vi "AlliGator Save-Load Settings.vi"(6 "Load(F)/Save (T)":bool, 8 "Error In":errorcluster, 10 "File Path":path, 11 "AlliGator Refnum in":refnum<vi>) -> (0 "Error Out":errorcluster, 2 "File Path out":path)   [LabVIEW 2021, in "AlliGator Settings.lvlib"]
doc: "Use this file to Save or Load AlliGator's settings to an ini file.\n\nIf the <B>File Path</B> input is left unconnected, the defaut ini file is used (overriding the current ini file).\n\nTo save settings in a user-specified location, either provide a valid path, or connect a \"Not a Path\" constant to the input. A File Dialog window will then open to allow the user to choose a path."
uses:
  AlliGator Settings.lvlib
  AlliGator Settings List.ctl
  <vilib>/Utility/sysdir.llb/System Directory Type.ctl
  97c900eb-8bb6-49ac-a854-86d526cd6a68.vi
  97c900eb-8bb6-49ac-a854-86d526cd6a68.vi/539bd7ec-d9e8-460f-a56d-a449b4a86a5e.vi
  Files/Files.lvlib
  <vilib>/Utility/config.llb/NI_LVConfig.lvlib
  <userlib>/_OpenG.lib/variantconfig/variantconfig.llb/openg_variant_configuration_file.lvlib
  Strings/Strings.lvlib
  Graphs/Graphs.lvlib
panel:
  in  "AlliGator Settings List":T1
  # "see the AlliGator License on the block diagram (Ctrl+E or Window:Show Block Diagram)"
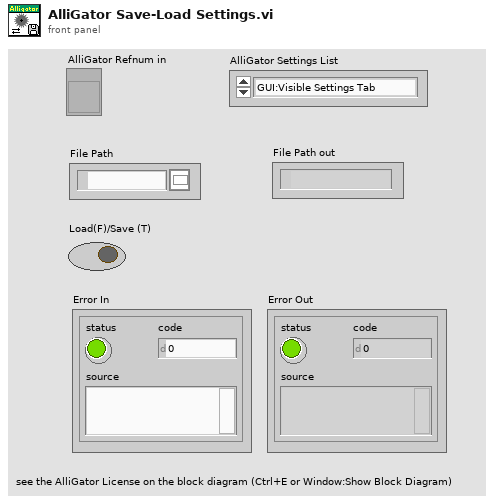
[diagram p1: front panel]
types:
  T1 = typedef "AlliGator Settings.lvlib/AlliGator Settings List.ctl" = enum16{"GUI:Visible Settings Tab", "GUI:Last Run Version", "Source Image:Use Image Histogram for Contrast", "Source Image:Low Count Pixels Rejection Options", "Source Image:High Count Pixels Rejection Options", "Source Image:Use Image Brightness", "Source Image:Blend Overlay with Image Background", "Source Image:Use Fixed ROI Diameter", "Source Image:ROI Diameter", "Source Image:ROI Center Color", "Source Image:Peak Threshold", "Source Image:Intensity Threshold", "Source Image:Image Binning Options", "Source Image:Image Smoothing Options", "Source Image:Image Histogram Active", "Source Image:Invert Binary Mask", "Source Image:Hot Pixel Removal", "Source Image:Overlay Analyzed ROI Center", "Source Image:Auto-Adjust Contrast", "Source Image:Histogram Lower Percentile", "Source Image:Histogram Upper Percentile", "Source Image:Save Source Image", "Source Image:Scale Bar Options", "Source Image:Image Resolution (Pixel Size)", "Source Image:Flatfield Correction", "Source Image:Show Dead Left Columns Correction", "Source Image:Dead Left Columns Correction", "Source Image:Image Pre-Processing Operations Order", "Data Information:Gate Width", "Data Information:Nanotime Gate Separation", "Data Information:Macrotime Gate Separation", "Data Information:Gate Step", "Data Information:# Gates", "Data Information:Gate Image Exposure", "Data Information:Gate Image Integration", "Data Information:Gates to Skip", "Data Information:Gates to Keep", "Data Information:Define Gates to", "Data Information:Channel Name", "Data Information:Available Channel Names", "Data Information:Channel Arithmetic", "Data Information:Background File Subtraction", "Data Information:Background File", "Data Information:Background Scaling Factor", "Data Information:Background Pile-up Correction", "Data Information:Background Pixel Well Capacity", "Data Information:Laser Period", "Data Information:SYNC Period", "Data Information:Pile-up Correction", "Data Information:Pixel Well Capacity", "Data Information:Dataset Scaling Factor", "Fluorescence Decay_Decay Pre-Processing:Reverse Gates", "Fluorescence Decay_Decay Pre-Processing:Verbose Decay Pre-Processing", "Fluorescence Decay_Decay Pre-Processing:Use Decay Pre-Processing", "Fluorescence Decay_Decay Pre-Processing:Background Subtraction", "Fluorescence Decay_Decay Pre-Processing:Background Definition Range", "Fluorescence Decay_Decay Pre-Processing:Baseline Subtraction Method", "Fluorescence Decay_Decay Pre-Processing:Decay Pre-Processing Operations Order", "Fluorescence Decay_Decay Pre-Processing:Smoothing Parameter", "Fluorescence Decay_Decay Pre-Processing:Shift Decay", "Fluorescence Decay_Decay Pre-Processing:Decay Shift Parameters", "Fluorescence Decay_Decay Pre-Processing:Fold Decay", "Fluorescence Decay_Decay Pre-Processing:# Folds", "Fluorescence Decay_Decay Pre-Processing:1-Normalize Decay", "Fluorescence Decay_Decay Pre-Processing:[0-1]-Normalize Decay", "Fluorescence Decay_Decay Pre-Processing:Smoothen Decay", "Fluorescence Decay_Decay Pre-Processing:Extrapolate Decay", "Fluorescence Decay_Decay Pre-Processing:Use Periodicity", "Fluorescence Decay_Decay Pre-Processing:Use Cursors", "Fluorescence Decay_Decay Pre-Processing:Tail Fraction", "Fluorescence Decay_Decay Pre-Processing:Head Fraction", "Fluorescence Decay_Decay Pre-Processing:Additional Points", "Fluorescence Decay_Decay Pre-Processing:Straighten Decay", "Fluorescence Decay_Decay Pre-Processing:Constant Background", "Fluorescence Decay_Decay Pre-Processing:Pixel-Normalize Decay", "Fluorescence Decay_Advanced Analysis:Extract IRF instead of Decay", "Fluorescence Decay_Advanced Analysis:IRF Extraction Options", "Fluorescence Decay_Advanced Analysis:IRF Optimization Options", "Fluorescence Decay_Advanced Analysis:Square Pulse Options", "Fluorescence Decay_Advanced Analysis:IRF Order", "Fluorescence Decay_Advanced Analysis:IRF Time Constants", "Fluorescence Decay_Advanced Analysis:Wavelet Analysis Options", "Fluorescence Decay_Advanced Analysis:Average Lifetime Options", "Fluorescence Decay_Fit Options:Fit Options", "Fluorescence Decay_Fit Options:Use Legacy Fitting Approach", "Fluorescence Decay_Fit Options:Use Data Information Laser Period", "Fluorescence Decay_Fit Parameters:Displayed Fit Parameters", "Fluorescence Decay_Fit Parameters:Fit Parameter Constraints", "Fluorescence Decay_Fit Parameters:Export Tabulated Results", "Fluorescence Decay_Fit Parameters:MLE Baseline Offset Type", "Fluorescence Decay_Fit Parameters:MLE Baseline Offset", "Fluorescence Decay_Fit Parameters:Guess Parameter Names", "Fluorescence Decay_Fit Parameters:Guess Parameter Values", "Fluorescence Decay_Fit Parameters:Guess Parameters Options", "Fluorescence Decay_Styles:Show Last Decay Only", "Fluorescence Decay_Styles:Decay Graph Color Array", "Fluorescence Decay:Decay Graph Active", "Fluorescence Decay Statistics:Min Peak Value", "Fluorescence Decay Statistics:Reject Low Decay Peak Pixels", "Fluorescence Decay Statistics:Reject High Decay Peak Pixels", "Fluorescence Decay Statistics:Max Peak Value", "Time Traces:Use File Timestamp", "Time Traces:Time Step", "Time Traces:Use Intensity Correction File", "Time Traces:Intensity Correction File", "Phasor Plot:Phasor Plot Smoothing Options", "Phasor Plot:Phasor Plot Size", "Phasor Plot:Phasor Plot Graphics Options", "Phasor Plot:Cumulative Phasor Plot", "Phasor Plot:Use Phasor Brightness", "Phasor Plot:Blend Overlay with Phasor Background", "Phasor Plot:Save Phasor Plot", "Phasor Plot:Show References", "Phasor Plot:Phasor Ratio Decay Range", "Phasor Plot:Exponential Fading", "Phasor Plot:Phasor Ratio Reference Colors", "Phasor Plot:Reference Radius", "Phasor Plot:Show Color Map Vertices", "Phasor Plot:Phasor Plot Active", "Phasor Plot:Phasor Ratio Color Map Type", "Phasor Plot:Phasor Ratio Color Map", "Phasor Plot:Phasor Ratio Display Range", "Phasor Plot:Selected Image ROI(s)", "Phasor Plot:All Image ROIs", "Phasor Plot:Selected Phasor Plot ROI(s)", "Phasor Plot:All Phasor Plot ROIs", "Phasor Plot:Phasor Ratio Color-Coded Quantity", "Phasor Plot:Store Phasor Harmonics", "Phasor Plot:Draw Reference Segment", "Phasor Plot:User-Defined Quantity", "Phasor Graph:Phasor Frequency", "Phasor Graph:Phasor Ratio Type", "Phasor Graph:Pixel-level Phasor Computation", "Phasor Graph:Save Phasor Graph", "Phasor Graph:Phasor Graph Active", "Phasor Graph:Phasor SDV Options", "Phasor Calibration:Use Backup Calibration if needed", "Phasor Graph:Define Shortest Lifetime as", "Phasor Calibration:Backup Calibration Type", "Phasor Calibration:Calibration Type", "Phasor Calibration:Calibration Lifetime", "Phasor Calibration:Calibration Map Algorithm", "Single-Exponential Phasor Locus (SEPL):Gate Parameters", "Single-Exponential Phasor Locus (SEPL):User-defined Gate", "Single-Exponential Phasor Locus (SEPL):User-defined IRF", "Single-Exponential Phasor Locus (SEPL):Phasor Parameters", "Single-Exponential Phasor Locus (SEPL):Decay & IRF Parameters", "Single-Exponential Phasor Locus (SEPL):Display Parameters", "Lifetime Analysis:Decay Analysis Parameters", "Lifetime Analysis:Lifetime Map Active", "Plugins:Python Settings", "Miscellaneous:Verbose Mode", "Miscellaneous:Beep after Script", "Miscellaneous:Saved Image File Format", "Miscellaneous:Exported Gate Image Settings", "Miscellaneous:Include Loading in Timing", "Miscellaneous:Verbose Settings Mode", "Miscellaneous:Histogram Options", "Miscellaneous:Beep on Error", "Miscellaneous:# Logical Processors Used", "Miscellaneous:ROI Description Max Characters", "Miscellaneous:Verbose Error Mode", "Miscellaneous:Transparent Mask Color"}
  T2 = typedef "System Directory Type.ctl" = i32
  T3 = typedef "NI_LVConfig.lvlib/Config Data RefNum.ctl" = refnum<k1>
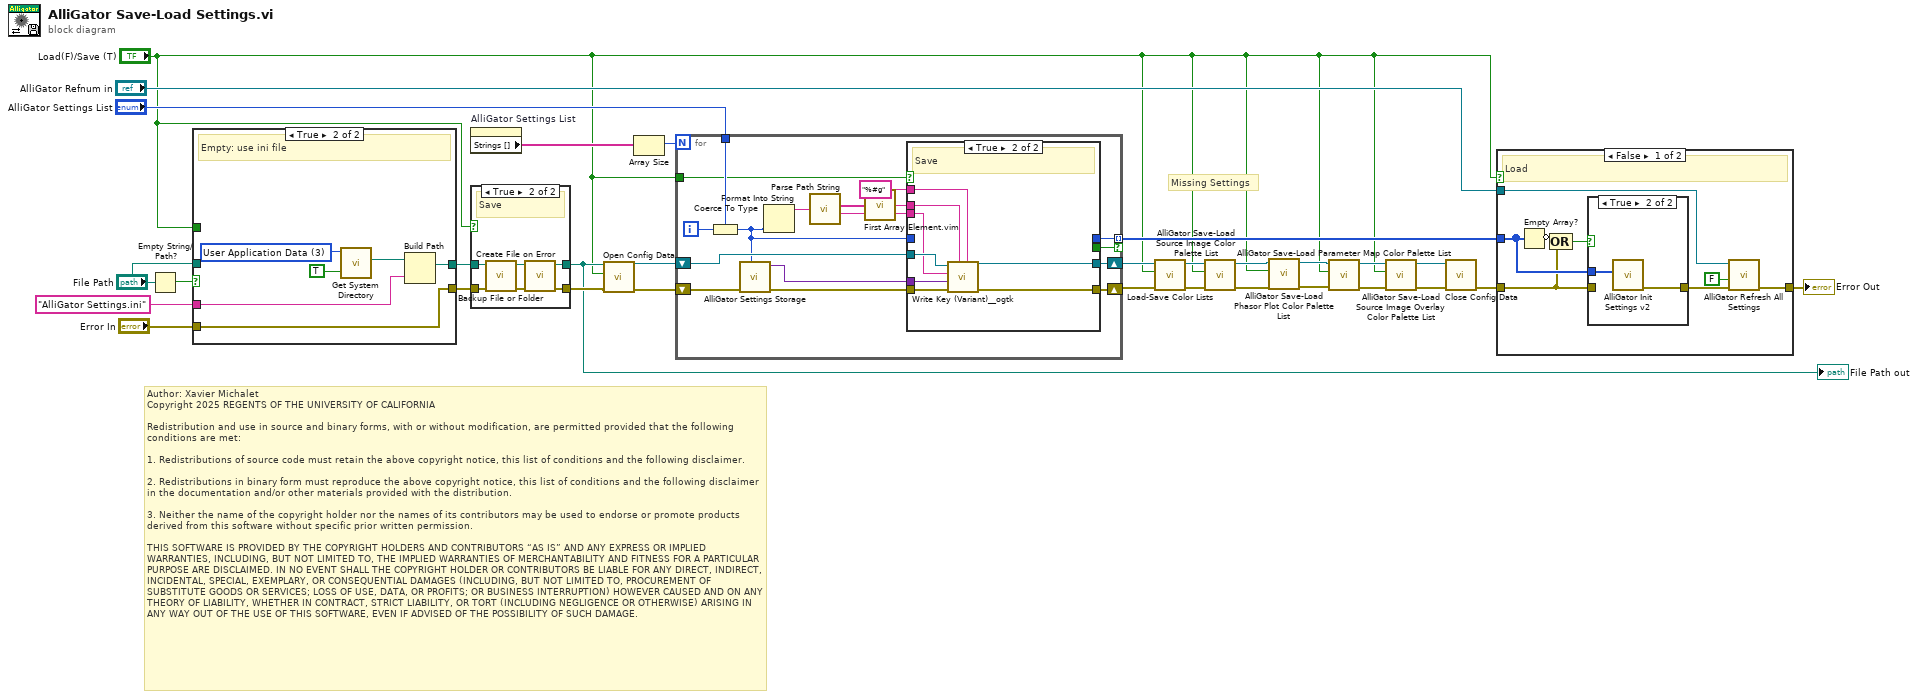
[diagram p0: block diagram]
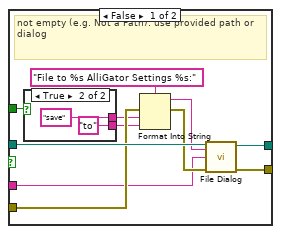
[diagram p2: hidden frame]
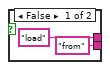
[diagram p3: hidden frame]
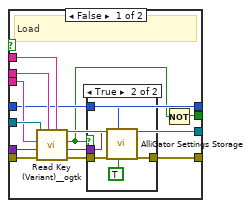
[diagram p6: hidden frame]
diagram:
  # "Author: Xavier Michalet\nCopyright 2025 REGENTS OF THE UNIVERSITY OF CALIFORNIA\n\nRedistribution and use in source and binary forms, with or without modification, are permitted provided that the following conditions are met:\n\n1. Redistributions of source code must retain the above copyright notice, this list of conditions and the following disclaimer.\n\n2. Redistributions in binary form must reproduce the above copyright notice, this list of conditions and the following disclaimer in the documentation and/or other materials provided with the distribution.\n\n3. Neither the name of the copyright holder nor the names of its contributors may be used to endorse or promote products derived from this software without specific prior written permission.\n\nTHIS SOFTWARE IS PROVIDED BY THE COPYRIGHT HOLDERS AND CONTRIBUTORS “AS IS” AND ANY EXPRESS OR IMPLIED WARRANTIES, INCLUDING, BUT NOT LIMITED TO, THE IMPLIED WARRANTIES OF MERCHANTABILITY AND FITNESS FOR A PARTICULAR PURPOSE ARE DISCLAIMED. IN NO EVENT SHALL THE COPYRIGHT HOLDER OR CONTRIBUTORS BE LIABLE FOR ANY DIRECT, INDIRECT, INCIDENTAL, SPECIAL, EXEMPLARY, OR CONSEQUENTIAL DAMAGES (INCLUDING, BUT NOT LIMITED TO, PROCUREMENT OF SUBSTITUTE GOODS OR SERVICES; LOSS OF USE, DATA, OR PROFITS; OR BUSINESS INTERRUPTION) HOWEVER CAUSED AND ON ANY THEORY OF LIABILITY, WHETHER IN CONTRACT, STRICT LIABILITY, OR TORT (INCLUDING NEGLIGENCE OR OTHERWISE) ARISING IN ANY WAY OUT OF THE USE OF THIS SOFTWARE, EVEN IF ADVISED OF THE POSSIBILITY OF SUCH DAMAGE."
  # "Missing Settings"
  n1 = Empty String/Path?(string/path="File Path") -> (empty?=w19:bool)
  n2 = case shown="True" w19 {
    tunnel: [w40 w48] -> w30
    tunnel: "Error In" -> [w35 w47]
    tunnel: [w39 w47] -> w17
    tunnel: "File Path" -> [w41 _]
    tunnel: "Load(F)/Save (T)" -> [w32 _]
    tunnel: "AlliGator Settings.ini" ("default name") -> [w31 w46]
    frame False {
      # "not empty (e.g. Not a Path): use provided path or dialog"
      n3 = case shown="True" w32 {
        tunnel: ["load" ("input 1") "save" ("input 1")] -> w34
        tunnel: ["from" ("input 2") "to" ("input 2")] -> w33
        frame False {
        }
        frame True {
        }
      }
      n4 = Format Into String(format string="File to %s AlliGator Settings %s:" ("prompt"), error in=w35, w34, w33) -> (resulting string=w37:string, error out=w36:errorcluster)  [unwired: 1 in]
      n5 = call "File Dialog"("start path"=w41, "prompt"=w37, "default name"=w31, "error in"=w36) -> ("selected path"=w40:path, "error out"=w39:errorcluster)  [unwired: 8 in, 2 out]
    }
    frame True {
      w49 = T2 3 items=["User Home"=0, "User Desktop"=1, "User Documents"=2, "User Application Data"=3, "User Preferences"=4, "User Temporary"=5, "Public Documents"=6, "Public Application Data"=7, "Public Preferences"=8, "Public Cache"=13, "System Core Libraries"=9, "System Installed Libraries"=10, "Application Files"=11, "Boot Volume Root"=12] ("system directory type")
      # "Empty: use ini file"
      n6 = call <vilib>:"Get System Directory.vi"("create directory if not found? (F)"=TRUE, "system directory type"=w49) -> ("system directory"=w50:path)  [unwired: 9 in]
      n7 = Build Path(base path=w50, name or relative path=w46) -> (appended path=w48:path)
    }
  }
  n8 = property on="AlliGator Settings List" class="Enum (strict)"() -> ("Strings []"=w25:string[])  [unwired: 2 in, 2 out]
  n9 = case shown="True" "Load(F)/Save (T)" {
    tunnel: w30 -> [w53 w59]
    tunnel: w17 -> [w52 w58]
    tunnel: [w53 w55] -> w12
    tunnel: [w52 w54] -> w29
    frame False {
      # "Laod"
    }
    frame True {
      # "Save"
      n10 = call "Backup File or Folder.vi"("error in (no error)"=w58, "File/Directory Path"=w59) -> ("error out"=w56:errorcluster, "File/Directory Path (dup)"=w57:path)  [unwired: 8 in]
      n11 = call "Create File on Error.vi"("error in (no error)"=w56, "File Path"=w57) -> ("error out"=w54:errorcluster, "File Path (dup)"=w55:path)  [unwired: 8 in]
    }
  }
  "File Path out" <- w12
  n12 = call <vilib>:"Open Config Data.vi"("error in (no error)"=w29, "create file if necessary (T)"="Load(F)/Save (T)", "configuration file path"=w12) -> ("error out"=w28:errorcluster, "refnum"=w27:T3)  [unwired: 6 in, 1 out]
  n13 = Array Size(array=w25) -> (size(s)=w24:i32)
  n14 = for {
    N: w24 -> [_]
    shift-right: [w69] -> w20
    shift-left: w28 -> [w75]
    shift-right: [w70] -> w21
    shift-left: w27 -> [w71]
    tunnel: "AlliGator Settings List" -> [w74]
    tunnel: "Load(F)/Save (T)" -> [w73]
    tunnel: [w61] -> w13 mode=indexing if=w60
    i -> [w76]
    n15 = Coerce To Type(0:w76, 1:w74) -> (2:w63:T1)
    n16 = call "AlliGator Settings Storage.vi"("AlliGator Settings List"=w63, "Error In"=w75) -> ("Error Out"=w72:errorcluster, "Variant Data out"=w68:variant)  [unwired: 8 in]
    n17 = Format Into String(w63) -> (resulting string=w67:string)  [unwired: 3 in, 1 out]
    n18 = call "Parse Path String.vi"("Path in"=w67) -> ("Folder Hierarchy"=w65:string[], "File/Folder"=w66:string)  [unwired: 4 in]
    n19 = call "First Array Element.vim"("Array"=w65) -> ("First Element"=w64:string)  [unwired: 8 in]
    n20 = case shown="True" w73 {
      tunnel: w71 -> [w89 w103]
      tunnel: [w86 w102] -> w70
      tunnel: w68 -> [w88 w99]
      tunnel: w72 -> [w87 w101]
      tunnel: [w82 w100] -> w69
      tunnel: w66 -> [w85 w98]
      tunnel: w64 -> [w84 w97]
      tunnel: w63 -> [w79 _]
      tunnel: "%#g" ("float number format") -> [w80 w96]
      tunnel: [w79 _] -> w61
      tunnel: [w78 _] -> w60
      frame False {
        # "Load"
        n21 = call <userlib>:"Read Key (Variant)__ogtk.vi"("format string (%;%f)"=w80, "section"=w84, "error in (no error)"=w87, "type"=w88, "key (optional)"=w85, "refnum"=w89) -> ("error out"=w83:errorcluster, "key-value"=w81:variant, "found?"=w77:bool, "refnum out"=w86:T3)  [unwired: 2 in]
        n22 = case shown="True" w77 {
          tunnel: w83 -> [w90 w95]
          tunnel: [w90 w94] -> w82
          tunnel: w79 -> [_ w92]
          tunnel: w81 -> [_ w91]
          frame False {
          }
          frame True {
            n23 = call "AlliGator Settings Storage.vi"("Get(F)/Set"=TRUE ("Get (F)/Set"), "AlliGator Settings List"=w92, "Error In"=w95, "Variant Data in"=w91) -> ("Error Out"=w94:errorcluster)  [unwired: 6 in, 1 out]
          }
        }
        n24 = Not(x=w77) -> (.not. x?=w78:bool)
      }
      frame True {
        # "Save"
        n25 = call <userlib>:"Write Key (Variant)__ogtk.vi"("float number format"=w96, "section"=w97, "error in (no error)"=w101, "key-value"=w99, "key (optional)"=w98, "refnum"=w103) -> ("error out"=w100:errorcluster, "refnum out"=w102:T3)  [unwired: 4 in]
      }
    }
  }
  n26 = call "Load-Save Color Lists.vi"("error in (no error)"=w20, "Load (F)/Save"="Load(F)/Save (T)", "ini File Refnum in"=w21) -> ("error out"=w10:errorcluster, "ini File Refnum out"=w11:T3)  [unwired: 7 in]
  n27 = call "AlliGator Save-Load Source Image Color Palette List.vi"("error in (no error)"=w10, "Load(F)/Save"="Load(F)/Save (T)", "Refnum in"=w11) -> ("error out"=w9:errorcluster, "Refnum out"=w8:T3)  [unwired: 7 in]
  n28 = call "AlliGator Save-Load Phasor Plot Color Palette List.vi"("error in (no error)"=w9, "Load(F)/Save"="Load(F)/Save (T)", "Refnum in"=w8) -> ("error out"=w6:errorcluster, "Refnum out"=w7:T3)  [unwired: 7 in]
  n29 = call "AlliGator Save-Load Parameter Map Color Palette List.vi"("error in (no error)"=w6, "Load(F)/Save"="Load(F)/Save (T)", "Refnum in"=w7) -> ("error out"=w5:errorcluster, "Refnum out"=w4:T3)  [unwired: 7 in]
  n30 = call "AlliGator Save-Load Source Image Overlay Color Palette List.vi"("error in (no error)"=w5, "Load(F)/Save"="Load(F)/Save (T)", "Refnum in"=w4) -> ("error out"=w1:errorcluster, "Refnum out"=w2:T3)  [unwired: 7 in]
  n31 = call <vilib>:"Close Config Data.vi"("error in (no error)"=w1, "refnum"=w2) -> ("error out"=w26:errorcluster)  [unwired: 8 in, 1 out]
  n32 = case shown="False" "Load(F)/Save (T)" {
    tunnel: w26 -> [w106 w115]
    tunnel: [w105 w115] -> w22
    tunnel: "AlliGator Refnum in" -> [w110 _]
    tunnel: w13 -> [w109 _]
    frame False {
      # "Load"
      n33 = Empty Array?(array=w109) -> (empty?=w108:bool)
      n34 = Compound Arithmetic op=OR(invert w108, w106) -> (w107:bool)
      n35 = case shown="True" w107 {
        tunnel: [w112 w114] -> w111
        tunnel: w109 -> [_ w113]
        tunnel: w106 -> [w112 _]
        frame False {
        }
        frame True {
          n36 = call "AlliGator Init Settings v2.vi"("Parameters to set to Default"=w113) -> ("error out"=w114:errorcluster)  [unwired: 10 in]
        }
      }
      n37 = call "AlliGator Refresh All Settings.vi"("Error In"=w111, "Verbose (T)"=FALSE, "VI Refnum in"=w110) -> ("Error Out"=w105:errorcluster)  [unwired: 8 in]
    }
    frame True {
      # "Save"
    }
  }
  "Error Out" <- w22
